vi "Message Address Global.vi"() -> ()   [LabVIEW 2009]
panel:
  in  "Addresses":T1(array[cluster])=[{"Module"="QCA", "Address"="127.0.0.1", "Port"=9326}, {"Module"="PDP", "Address"="127.0.0.1", "Port"=9327}, {"Module"="TEB", "Address"="127.0.0.1", "Port"=9328}, {"Module"="TCL", "Address"="127.0.0.1", "Port"=9329}, {"Module"="OLA", "Address"="127.0.0.1", "Port"=9330}]
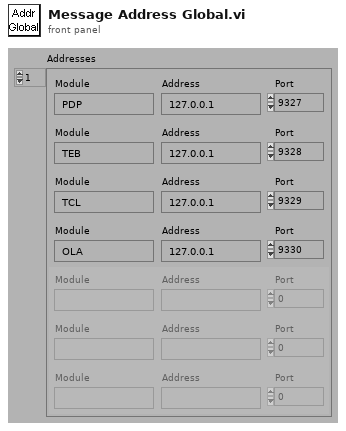
[diagram p1: front panel]
types:
  T1 = cluster{"Module":string, "Address":string, "Port":u16}[]
diagram:
